vi "Update_e_t.vi"(7 "Rest":bool, 8 "input valid":bool=TRUE, 11 "e(t)":fxp<+/-,32,4>) -> (0 "output valid":bool, 2 "e(t-1)-e(t-2)":fxp<+/-,32,4>, 3 "e(t)-e(t-1)":fxp<+/-,32,4>)   [LabVIEW 2013]
uses:
  <vilib>/rvi/FXPMathLib/FxpSub/XNode/nifxpmath_Sub.xnode
  <vilib>/rvi/FXPMathLib/sim/FxpSim.dll
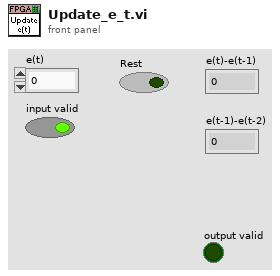
[diagram p1: front panel]
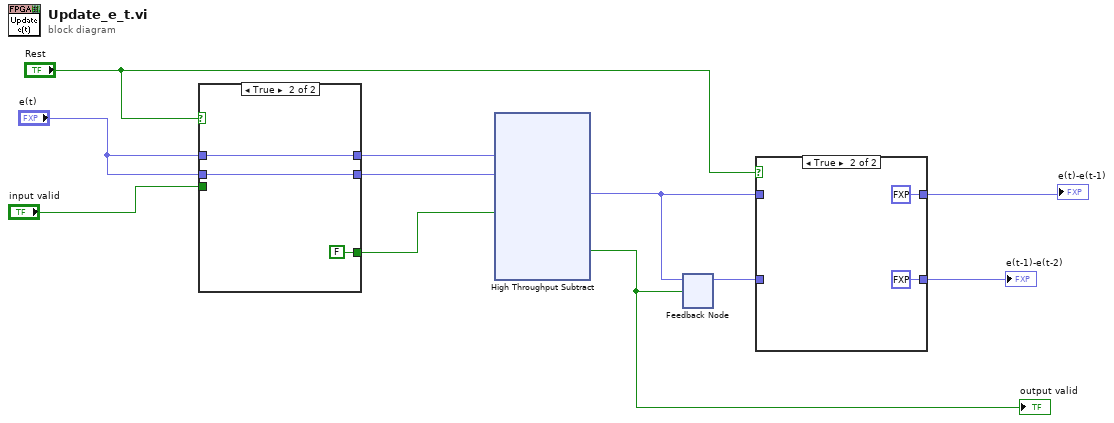
[diagram p0: block diagram]
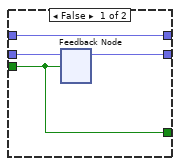
[diagram p3: hidden frame]
diagram:
  n1 = case shown="True" "Rest" {
    tunnel: "e(t)" -> [w15 w17]
    tunnel: [w14 w17] -> w11
    tunnel: "input valid" -> [w12 _]
    tunnel: "e(t)" -> [w13 w18]
    tunnel: [w13 w18] -> w7
    tunnel: [w12 FALSE ("input valid")] -> w6
    frame False {
      n2 = feedback #1() -> (w14:fxp<+/-,32,4>)  [unwired: 1 in]
      n3 = feedback-in #1(w15, w12) -> ()
    }
    frame True {
    }
  }
  n4 = xnode "High Throughput Subtract"("x"=w7, "y"=w11, "input valid"=w6) -> ("x-y"=w4:fxp<+/-,32,4>, "output valid"=w10:bool)  [unwired: 1 in, 1 out]
  "output valid" <- w10
  n5 = feedback #2() -> (w3:fxp<+/-,32,4>)  [unwired: 1 in]
  n6 = feedback-in #2(w4, w10) -> ()
  n7 = case shown="True" "Rest" {
    tunnel: w4 -> [w20 _]
    tunnel: w3 -> [w19 _]
    tunnel: [w20 fxp<+/-,32,4> 0.0 ("x-y")] -> w2
    tunnel: [w19 fxp<+/-,32,4> 0.0 ("x-y")] -> w1
    frame False {
    }
    frame True {
    }
  }
  "e(t)-e(t-1)" <- w2
  "e(t-1)-e(t-2)" <- w1
